vi "KITSAT_반틈.vi"() -> ()   [LabVIEW 2011]
uses:
  <vilib>/Math Plots/3D Math Plots/3D Stem/3D Stem XCtrl/3D Stem.xctl
  <vilib>/Utility/file.llb/Write To Spreadsheet File (string).vi
  <vilib>/Math Plots/3D Math Plots/3D Stem/3D Stem Datatype/Public/Plot Helper (Vector).vi
  <vilib>/vision/NI_Vision_Development_Module.lvlib
  <vilib>/Math Plots/3D Math Plots/3D Stem/3D Stem Datatype/3D Stem Datatype.lvclass
panel:
  out "낙하 중 현재 위치":refnum<class "3D Plot Datatype.lvclass">[](xcontrol)
  in  "Stop 2":bool
  out "경고등":bool
  out "공기 오염도":i32(graph)
  out "습 도":dbl(graph)
  out "Brightness Color (light temprature)":T1(plugin-control)
  out "Origin + Threshold":T1(plugin-control)
  in  "Image Type 5":T2 items=["Grayscale (U8)", "Grayscale (I16)", "Grayscale (SGL)", "Complex (CSG)", "RGB (U32)", "HSL (U32)", "RGB (U64)", "Grayscale (U16)"]
  out "Labeled Image (Threshold)":T1(plugin-control)
  in  "Connectivity":bool
  in  "Image Type 2":T2 items=["Grayscale (U8)", "Grayscale (I16)", "Grayscale (SGL)", "Complex (CSG)", "RGB (U32)", "HSL (U32)", "RGB (U64)", "Grayscale (U16)"]
  in  "Stop":bool
  # "KITSAT IMAGE PROCESSING PROGRAM"
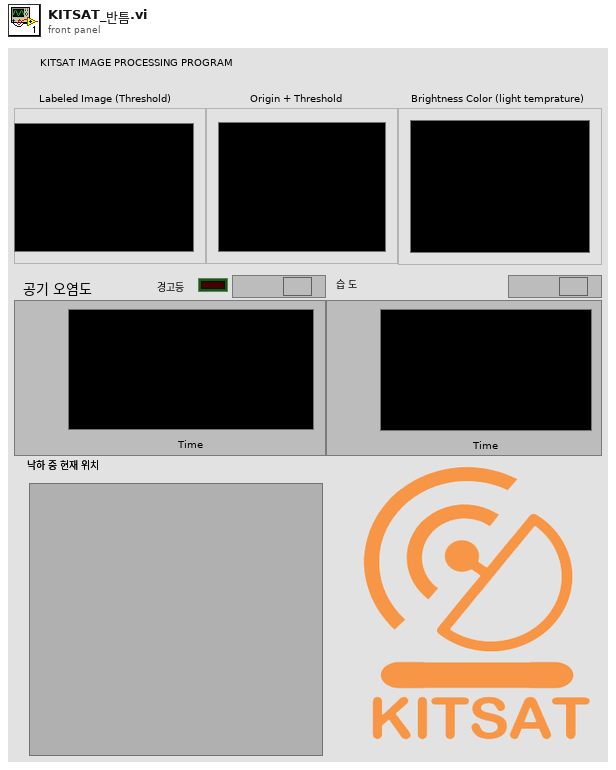
[diagram p1: front panel]
types:
  T1 = typedef "IMAQ Image.ctl" = refnum<image>
  T2 = typedef "Image Type" = u32
  T3 = typedef "AviRefnum.ctl" = refnum<k1>
  T4 = cluster{"Brightness":sgl, "Contrast":sgl, "Gamma":sgl}
  T5 = enum32{"AutoM", "Close", "Dilate", "Erode", "Gradient", "Gradient out", "Gradient in", "Hit miss", "Open", "PClose", "POpen", "Thick", "Thin"}
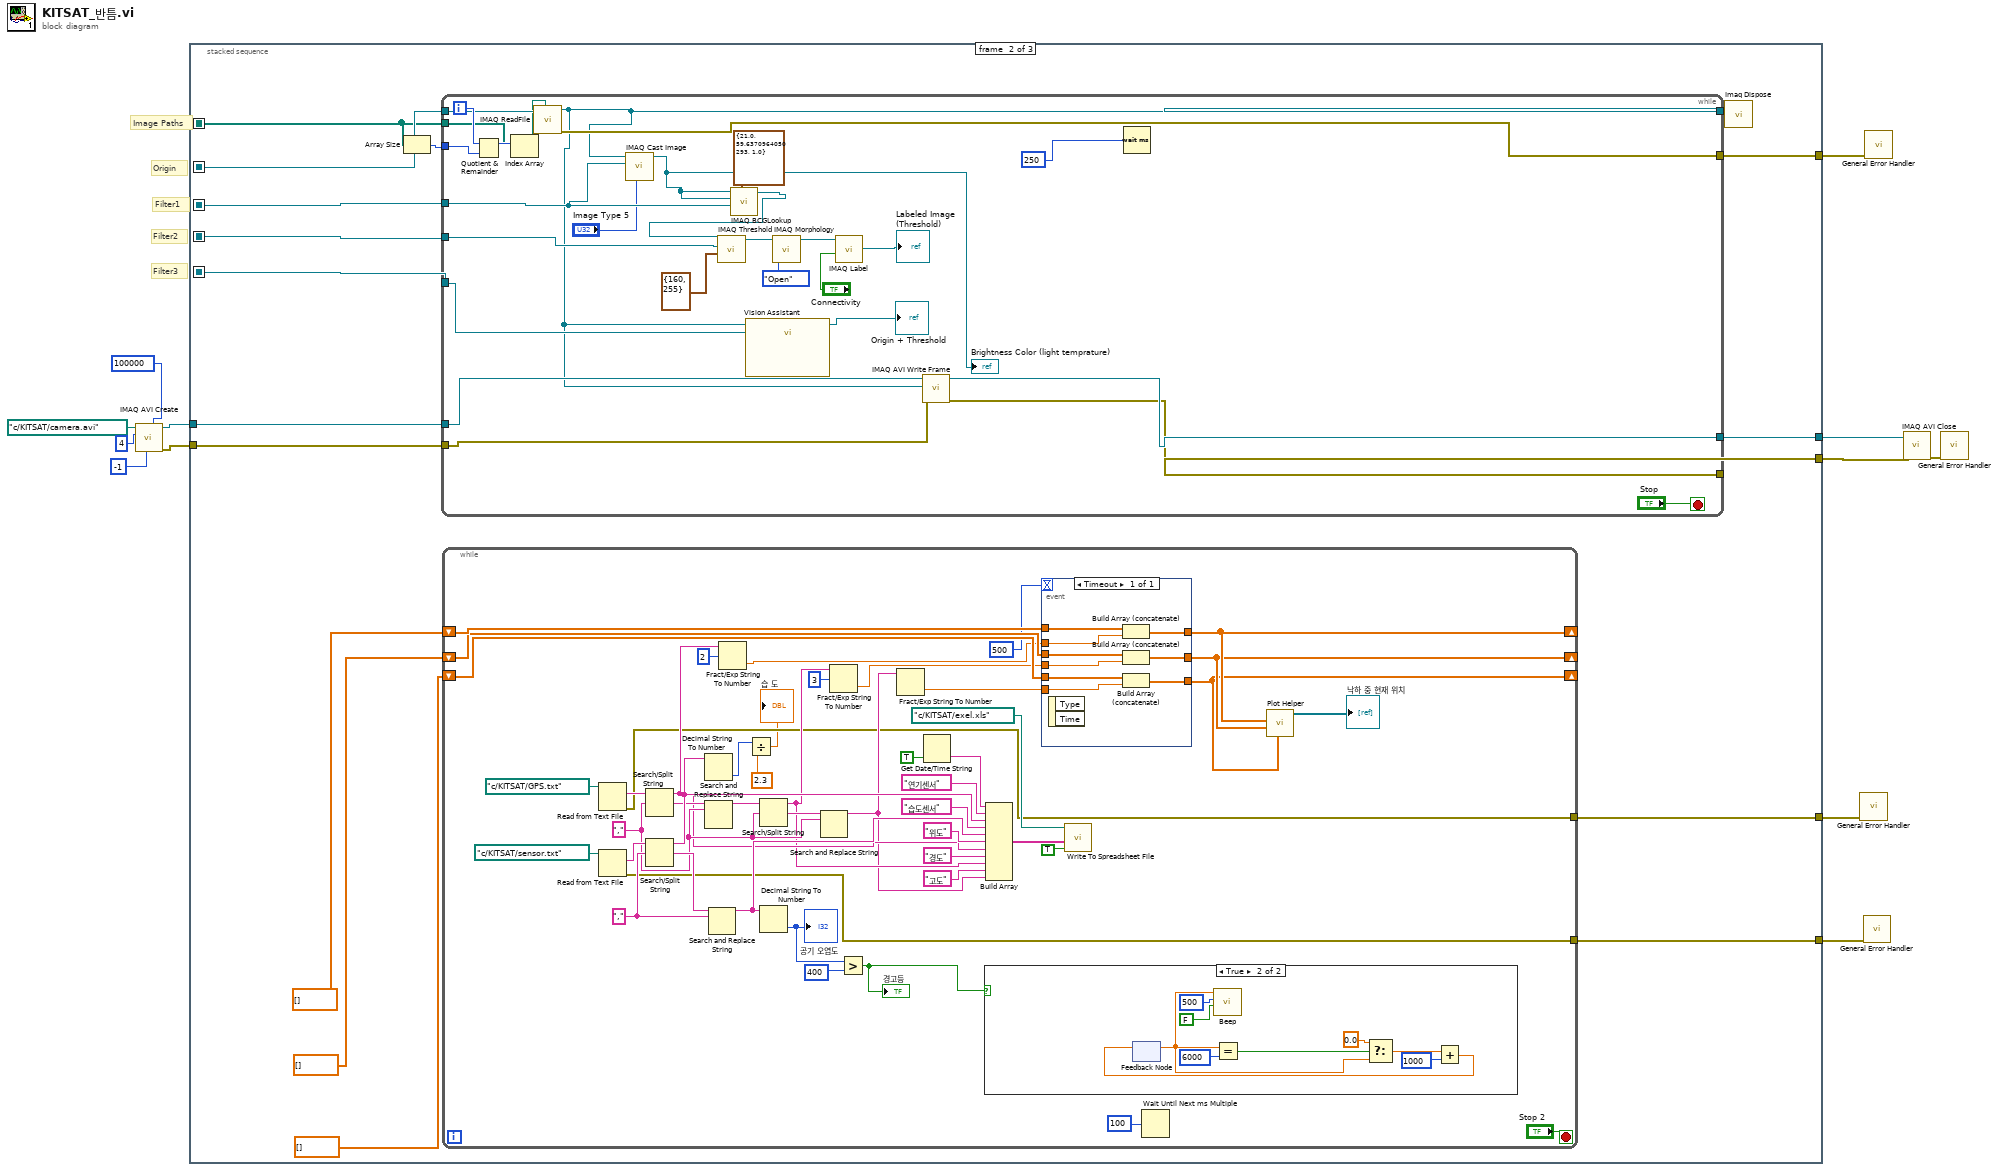
[diagram p0: block diagram]
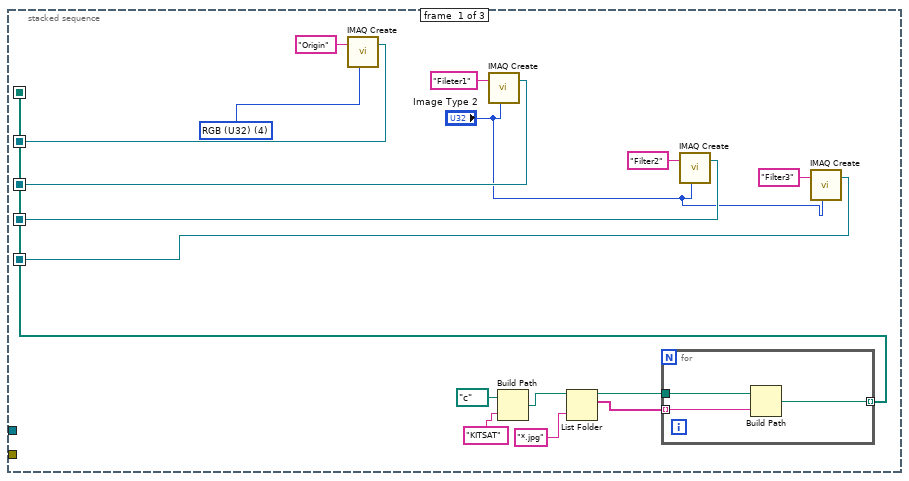
[diagram p2: hidden frame]
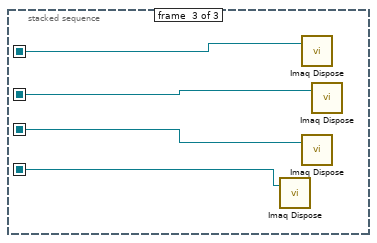
[diagram p4: hidden frame]
diagram:
  # "Filter3"
  # "Filter2"
  # "Filter1"
  # "Image Paths"
  # "Origin"
  n1 = call "IMAQ AVI Create"("Max Data Size"=u32 100000, "quality"=-1, "Frames Per Second"=u32 4, "AVI Path"=path "c:/KITSAT/camera.avi") -> ("error out"=w9:errorcluster, "Avi Refnum"=w10:T3)  [unwired: 6 in]
  n2 = stacked-sequence {
    seq-local: [w27 _ _] -> [_ w49 w147]
    seq-local: [w22 _ _] -> [_ w48 _]
    seq-local: [w18 _ _] -> [_ w46 w146]
    seq-local: [w17 _ _] -> [_ w45 w145]
    seq-local: [w15 _ _] -> [_ w44 w144]
    tunnel: w10 -> [_ w42 _]
    tunnel: [_ w41 _] -> w4
    tunnel: w9 -> [_ w40 _]
    tunnel: [_ w39 _] -> w5
    tunnel: [_ w35 _] -> w3
    tunnel: [_ w34 _] -> w2
    tunnel: [_ w33 _] -> w1
    frame #0 {
      w13 = u32 4 items=["Grayscale(U8)", "Grayscale(I16)", "Grayscale(SGL)", "Complex(CSG)", "RGB (U32)", "HSL (U32)", "RGB (U64)", "Grayscale (U16)"] ("Image Type(RGB)")
      n3 = call "IMAQ Create"("Image Name"="Origin", "Image Type"=w13) -> ("New Image"=w27:T1)  [unwired: 2 in, 2 out]
      n4 = call "IMAQ Create"("Image Name"="Fileter1", "Image Type"="Image Type 2") -> ("New Image"=w18:T1)  [unwired: 2 in, 2 out]
      n5 = Build Path(base path=path "c:/", name or relative path="KITSAT") -> (appended path=w26:path)
      n6 = List Folder(path=w26, pattern="*.jpg") -> (path out=w25:path, filenames=w24:string[])  [unwired: 1 in, 3 out]
      n7 = for {
        tunnel: w24 -> [w31] mode=indexing
        tunnel: w25 -> [w32]
        tunnel: [w30] -> w22 mode=indexing
        n8 = Build Path(base path=w32, name or relative path=w31) -> (appended path=w30:path)
      }
      n9 = call "IMAQ Create"("Image Name"="Filter2", "Image Type"="Image Type 2") -> ("New Image"=w17:T1)  [unwired: 2 in, 2 out]
      n10 = call "IMAQ Create"("Image Name"="Filter3", "Image Type"="Image Type 2") -> ("New Image"=w15:T1)  [unwired: 2 in, 2 out]
    }
    frame #1 {
      n11 = Array Size(array=w48) -> (size(s)=w47:i32)
      n12 = while {
        tunnel: w49 -> [w139]
        tunnel: w48 -> [w140]
        tunnel: w47 -> [w142]
        tunnel: w46 -> [w127]
        tunnel: w45 -> [w130]
        tunnel: w44 -> [w125]
        tunnel: [w116] -> w43
        tunnel: w42 -> [w123]
        tunnel: [w122] -> w41
        tunnel: w40 -> [w121]
        tunnel: [w119] -> w39
        tunnel: [w117] -> w33
        i -> [w143]
        stop <- "Stop" stop-if-true
        n13 = Quotient & Remainder(x=w143, y=w142) -> (x-y*floor(x/y)=w141:i32)  [unwired: 1 out]
        n14 = Index Array(array=w140, index=w141) -> (element=w138:path)
        n15 = call "IMAQ ReadFile"("File Path"=w138, "Image"=w139) -> ("error out"=w117:errorcluster, "Image Out"=w116:T1)  [unwired: 3 in, 5 out]
        n16 = call "IMAQ Cast Image"("Image Type"="Image Type 5", "Image Dst"=w127, "Image Src"=w116) -> ("Image Dst Out"=w120:T1)  [unwired: 7 in, 1 out]
        "Brightness Color (light temprature)" <- w120
        n17 = call "IMAQ BCGLookup"("Image Src"=w120, "BCG Values"=T4 {"Brightness"=21.0, "Contrast"=59.637096, "Gamma"=1.0}, "Image Mask"=w120, "Image Dst"=w127) -> ("Image Dst Out"=w131:T1)  [unwired: 3 in, 1 out]
        n18 = call "IMAQ Threshold"("Range"=cluster{i32, i32} {160, 255} ("Threshold"), "Image Dst"=w130, "Image Src"=w131) -> ("Image Dst Out"=w134:T1)  [unwired: 3 in, 5 out]
        n19 = call "Vision Assistant"("Image In"=w116, "Image Dst"=w125) -> ("Image Out"=→"Origin + Threshold":T1)  [unwired: 24 in, 1 out]
        n20 = call "IMAQ Morphology"("Operation"=T5."Open", "Image Src"=w134) -> ("Image Dst Out"=w132:T1)  [unwired: 5 in, 4 out]
        n21 = call "IMAQ Label"("Connectivity 4/8 (8)"="Connectivity", "Image Src"=w132) -> ("Image Dst Out"=→"Labeled Image (Threshold)":T1)  [unwired: 2 in, 2 out]
        n22 = call "IMAQ AVI Write Frame"("error in (no error)"=w121, "Image"=w116, "Avi Refnum"=w123) -> ("error out"=w119:errorcluster, "Avi Refnum (duplicate)"=w122:T3)  [unwired: 7 in]
        n23 = Wait (ms)(milliseconds to wait=u32 250) -> ()  [unwired: 1 out]
      }
      n24 = while {
        shift-right: [w76] -> _
        shift-left: dbl[] [] -> [w80]
        shift-right: [w75] -> _
        shift-left: dbl[] [] -> [w79]
        shift-right: [w74] -> _
        shift-left: dbl[] [] -> [w78]
        tunnel: [w54] -> w35
        tunnel: [w53] -> w34
        stop <- "Stop 2" stop-if-true
        w68 = ","
        w81 = ","
        n25 = Read from Text File(file (use dialog)=path "c:/KITSAT/GPS.txt") -> (text=w73:string, error out=w54:errorcluster)  [unwired: 3 in, 2 out]
        n26 = Read from Text File(file (use dialog)=path "c:/KITSAT/sensor.txt") -> (text=w97:string, error out=w53:errorcluster)  [unwired: 3 in, 2 out]
        n27 = Search/Split String(string=w73, search string/char (-)=w68) -> (substring before match=w57:string, match + rest of string=w71:string)  [unwired: 1 in, 1 out]
        n28 = Search/Split String(string=w97, search string/char (-)=w81) -> (substring before match=w92:string, match + rest of string=w96:string)  [unwired: 1 in, 1 out]
        n29 = Decimal String To Number(string=w92) -> (number=w50:i32)  [unwired: 2 in, 1 out]
        n30 = Search and Replace String(input string=w71, search string=w68) -> (result string=w70:string)  [unwired: 6 in, 3 out]
        n31 = Search and Replace String(input string=w96, search string=w81) -> (result string=w86:string)  [unwired: 1 in, 8 out]
        n32 = Fract/Exp String To Number(string=w57, offset=2) -> (number=w65:dbl)  [unwired: 2 in, 1 out]
        n33 = Divide(x=w50, y=2.3) -> (x/y=→"습 도":dbl)
        n34 = Search/Split String(string=w70, search string/char (-)=w68) -> (substring before match=w56:string, match + rest of string=w69:string)  [unwired: 1 in, 1 out]
        n35 = Decimal String To Number(string=w86) -> (number=w95:i32)  [unwired: 2 in, 1 out]
        "공기 오염도" <- w95
        n36 = Search and Replace String(input string=w69, search string=w68) -> (result string=w55:string)  [unwired: 6 in, 3 out]
        n37 = Fract/Exp String To Number(string=w56, offset=3) -> (number=w64:dbl)  [unwired: 2 in, 1 out]
        n38 = Greater?(x=w95, y=400) -> (0:w93:bool)
        "경고등" <- w93
        n39 = Fract/Exp String To Number(string=w55) -> (number=w63:dbl)  [unwired: 3 in, 1 out]
        n40 = Get Date/Time String(want seconds? (F)=TRUE) -> (time string=w85:string)  [unwired: 2 in, 1 out]
        n41 = case shown="True" w93 {
          frame False {
          }
          frame True {
            n42 = feedback #1() -> (w108:dbl)  [unwired: 1 in]
            n43 = call <vilib>:"Beep.vi"("use system alert? (T)"=FALSE, "duration (msec)"=u32 500, "frequency (Hz)"=w108) -> ()  [unwired: 9 in]
            n44 = Equal?(x=w108, y=6000) -> (x = y?=w110:bool)
            n45 = Select(t=0.0, s=w110, f=w108) -> (s? t:f=w107:dbl)
            n46 = Add(x=w107, y=1000) -> (x+y=w113:dbl)
            n47 = feedback-in #1(w113) -> ()
          }
        }
        n48 = Build Array(w85, "연기센서", w92, "습도센서", w86, "위도", w57, "경도", w56, "고도", w55) -> (w88:string[])
        n49 = event shown="[0] Timeout" {
          selector: _ -> [_]
          dyn-events: _ -> [_]
          timeout: 500 -> [_]
          tunnel: w80 -> [w106]
          tunnel: [w105] -> w76
          tunnel: w79 -> [w104]
          tunnel: [w103] -> w75
          tunnel: w78 -> [w102]
          tunnel: [w101] -> w74
          tunnel: w65 -> [w100]
          tunnel: w64 -> [w99]
          tunnel: w63 -> [w98]
          event Timeout {
            n50 = event-data() -> ()  [unwired: 1 in, 2 out]
            n51 = Build Array (concatenate)(w106, w100) -> (w105:dbl[])
            n52 = Build Array (concatenate)(w104, w99) -> (w103:dbl[])
            n53 = Build Array (concatenate)(w102, w98) -> (w101:dbl[])
          }
        }
        n54 = call-poly <vilib>:"Write To Spreadsheet File.vi"("append to file? (new file:F)"=TRUE, "1D data"=w88, "file path (dialog if empty)"=path "c:/KITSAT/exel.xls") -> ()  [unwired: 5 in, 1 out]
        n55 = Wait Until Next ms Multiple(millisecond multiple=u32 100 ("ms 배수")) -> ()  [unwired: 1 out]
        n56 = call-poly <vilib>:"Plot Helper.vi"("z vector"=w74, "y vector"=w75, "x vector"=w76) -> ("3D Plot lvclass Array out"=→"낙하 중 현재 위치":refnum<class "3D Plot Datatype.lvclass">[])  [unwired: 3 in, 5 out]
      }
      n57 = call "Imaq Dispose"("Image"=w43) -> ()  [unwired: 2 in, 4 out]
    }
    frame #2 {
      n58 = call "Imaq Dispose"("Image"=w144) -> ()  [unwired: 2 in, 4 out]
      n59 = call "Imaq Dispose"("Image"=w147) -> ()  [unwired: 2 in, 4 out]
      n60 = call "Imaq Dispose"("Image"=w145) -> ()  [unwired: 2 in, 4 out]
      n61 = call "Imaq Dispose"("Image"=w146) -> ()  [unwired: 2 in, 4 out]
    }
  }
  n62 = call <vilib>:"General Error Handler.vi"("error in (no error)"=w3) -> ()  [unwired: 10 in, 5 out]
  n63 = call <vilib>:"General Error Handler.vi"("error in (no error)"=w2) -> ()  [unwired: 10 in, 5 out]
  n64 = call <vilib>:"General Error Handler.vi"("error in (no error)"=w1) -> ()  [unwired: 10 in, 5 out]
  n65 = call "IMAQ AVI Close"("error in (no error)"=w5, "Avi Refnum"=w4) -> ("error out"=w8:errorcluster)  [unwired: 9 in]
  n66 = call <vilib>:"General Error Handler.vi"("error in (no error)"=w8) -> ()  [unwired: 10 in, 5 out]
